vi "Data_Logger_Main.vi"() -> ()   [LabVIEW 2025]
uses:
  <vilib>/Utility/file.llb/Write Delimited Spreadsheet (DBL).vi
panel:
  in  "Validation_save_path":path
  in  "Train_save_path":path
  in  "Road Tilt":dbl(knob) scale=-15.0..15.0
  in  "Driving Style":u32(knob) scale=0.0..2.0
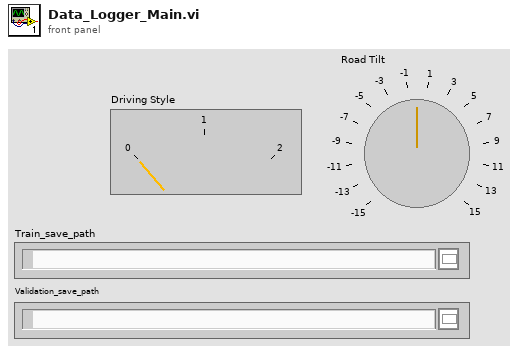
[diagram p1: front panel]
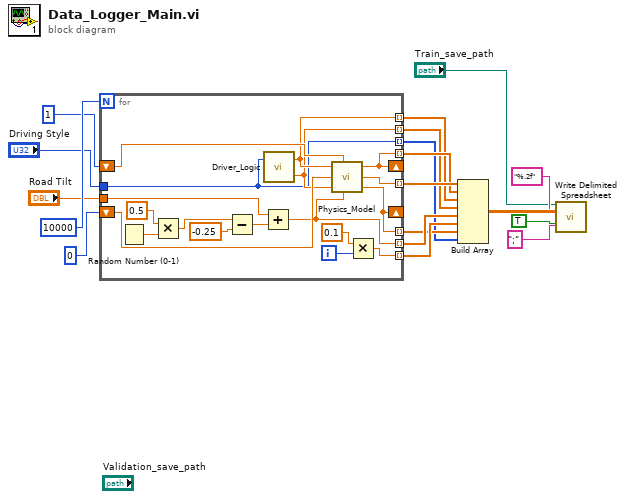
[diagram p0: block diagram]
diagram:
  n1 = for {
    N: 10000 -> [_]
    shift-right: [w21] -> _
    shift-left: 0 -> [w30]
    shift-right: [w26] -> _
    shift-left: 1 -> [w31]
    tunnel: "Road Tilt" -> [w33]
    tunnel: "Driving Style" -> [w20]
    tunnel: [w27] -> w13 mode=indexing
    tunnel: [w26] -> w12 mode=indexing
    tunnel: [w25] -> w11 mode=indexing
    tunnel: [w24] -> w10 mode=indexing
    tunnel: [w23] -> w9 mode=indexing
    tunnel: [w22] -> w8 mode=indexing
    tunnel: [w21] -> w7 mode=indexing
    tunnel: [w20] -> w6 mode=indexing
    i -> [w29]
    n2 = Random Number (0-1)() -> (number: 0 to 1=w36:dbl)
    n3 = Multiply(x=0.5, y=w36) -> (x*y=w35:dbl)
    n4 = Subtract(x=w35, y=-0.25) -> (x-y=w32:dbl)
    n5 = Add(x=w33, y=w32) -> (x+y=w23:dbl)
    n6 = call "Driver_Logic.vi"("Driving Style"=w20) -> ("Brake_Out"=w24:dbl, "Throttle_Out"=w25:dbl)  [unwired: 1 in]
    n7 = call "Physics_Model.vi"("Throttle[%]"=w25, "prev_gear"=w31, "Prev_Speed[km/h]"=w30, "Brake[%]"=w24, "Tilt_sensor"=w23) -> ("Speed_New"=w26:dbl, "RPM"=w27:dbl, "new_gear"=w21:dbl)
    n8 = Multiply(x=0.1, y=w29) -> (x*y=w22:dbl)
  }
  n9 = Build Array(w13, w12, w11, w10, w9, w8, w7, w6) -> (w5:dbl[][])
  n10 = call-poly <vilib>:"Write Delimited Spreadsheet.vi"("file path (dialog if empty)"="Train_save_path", "format (%.3f)"="%.2f", "2D data"=w5, "append to file? (new file:F)"=TRUE, "delimiter (\\t)"=";" ("delimiter (\\t)")) -> ()  [unwired: 9 in, 2 out]
